vi "Input File Step Iterator.vi"(6 "error in (no error)":errorcluster, 8 "LBCB Input Files":path[](array[path]), 9 "Input File Step Actions":T4) -> (0 "error out":errorcluster, 1 "End of Input File":bool, 2 "Last Step":i32, 3 "Next Step":T1)   [LabVIEW 2009]
uses:
  Input File Step Actions.ctl
  MixedMode/Load Step.ctl
  MixedMode/Messages/Target.ctl
  Data Access Objects/Metadata/LBCB Number.ctl
panel:
  out "Current Step":i32
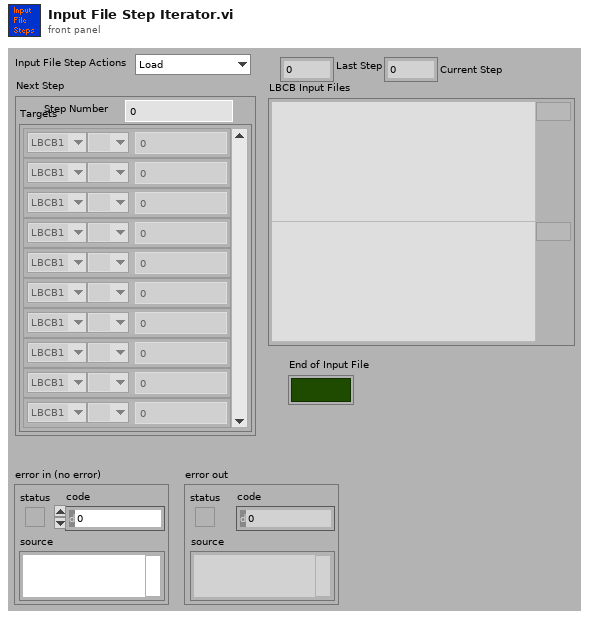
[diagram p1: front panel]
types:
  T1 = typedef "Load Step.ctl" = cluster{"Step Number":u32, "Targets":T2[]}
  T2 = typedef "Target.ctl" = cluster{"LBCB Number":T3, "DOF Vectors":enum16{" ", "Dx", "Dy", "Dz", "Rx", "Ry", "Rz", "Fx", "Fy", "Fz", "Mx", "My", "Mz"}, "Amount":dbl}
  T3 = typedef "LBCB Number.ctl" = enum16{"LBCB1", "LBCB2"}
  T4 = typedef "Input File Step Actions.ctl" = enum16{"Load", "Next Step", "Reset", "Get Step", "Backup"}
  T5 = enum16{"Init", "Set Step", "Set Correction Step", "Set Step String", "Get Step String"}
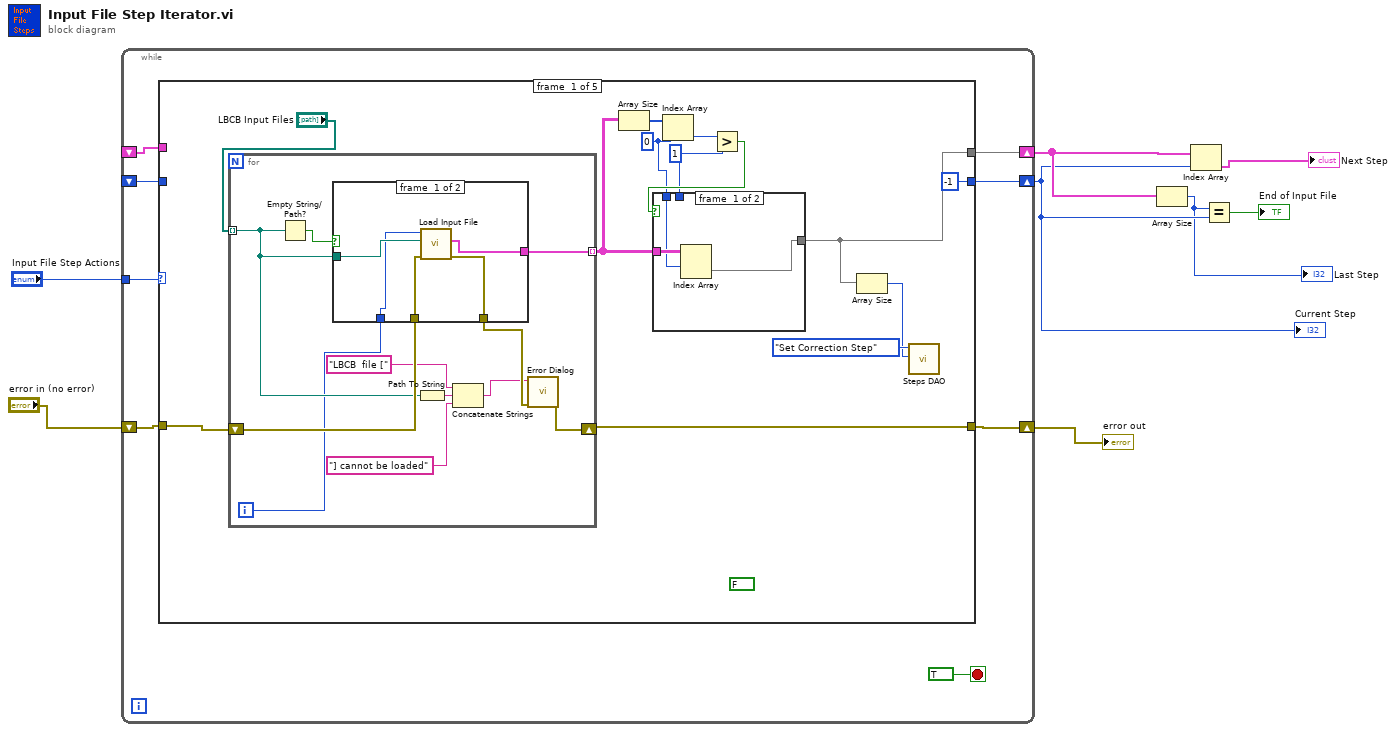
[diagram p0: block diagram]
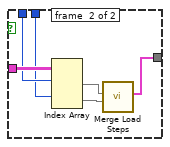
[diagram p2: hidden frame]
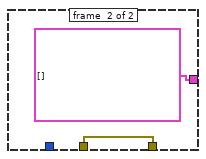
[diagram p3: hidden frame]
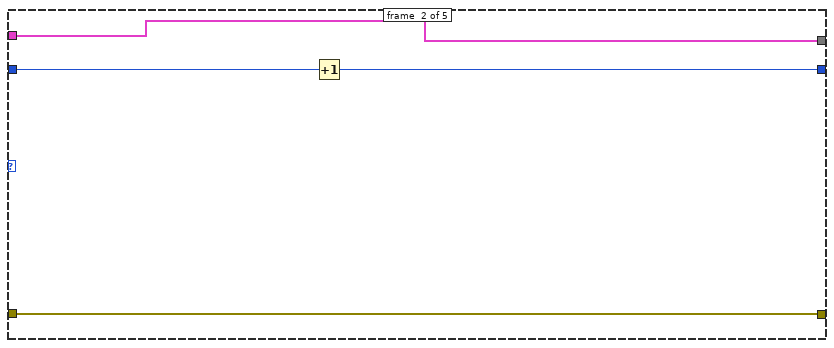
[diagram p4: hidden frame]
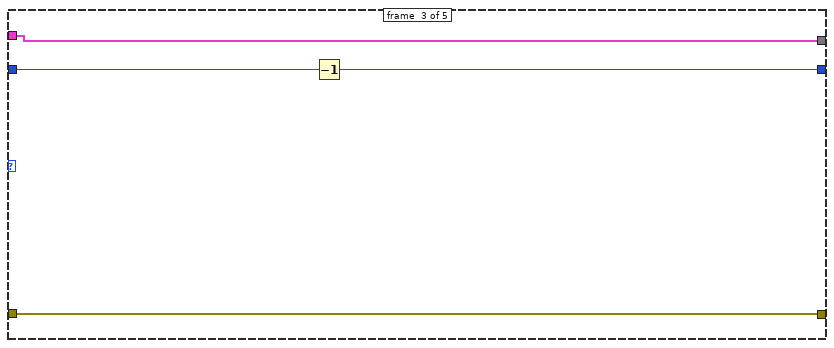
[diagram p5: hidden frame]
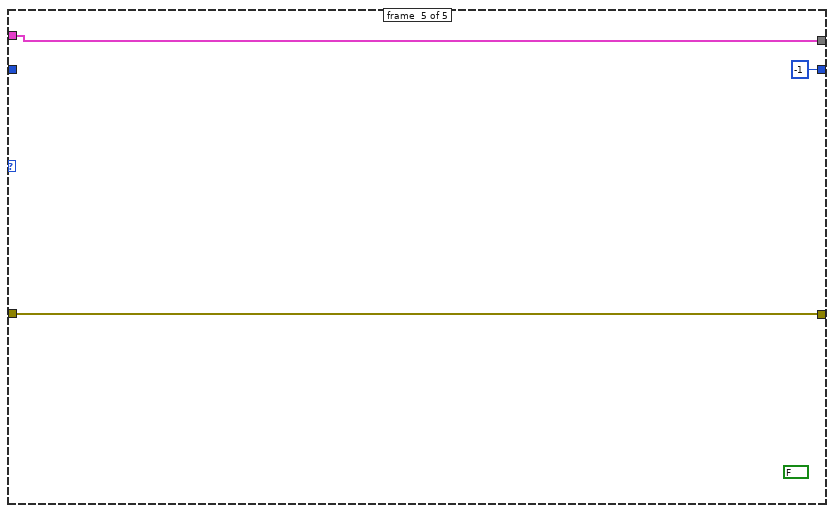
[diagram p7: hidden frame]
diagram:
  n1 = while {
    tunnel: "Input File Step Actions" -> [w15]
    shift-right: [w13] -> w6
    shift-left: "error in (no error)" -> [w14]
    shift-right: [w12] -> w5
    shift-left: _ -> [w10]
    shift-right: [w11] -> w4
    shift-left: _ -> [w9]
    stop <- TRUE stop-if-true
    n2 = case shown="\"Load\"" w15 {
      tunnel: w14 -> [w29 w59 w63 w67 w69]
      tunnel: [w27 w59 w63 w67 w69] -> w13
      tunnel: [w18 w57 w62 w66 w70] -> w12
      tunnel: [-1 w58 w61 w65 -1] -> w11
      tunnel: w10 -> [_ w57 w62 w66 w70]
      tunnel: w9 -> [_ w60 w64 w65 _]
      frame #0 {
        (unwired) FALSE
        w21 = 1 ("y")
        w22 = 0 ("index")
        n3 = for {
          tunnel: "LBCB Input Files" -> [w42] mode=indexing
          shift-right: [w41] -> w27
          shift-left: w29 -> [w48]
          tunnel: [w40] -> w23 mode=indexing
          i -> [w39]
          n4 = Empty String/Path?(string/path=w42) -> (empty?=w49:bool)
          n5 = case shown="False" w49 {
            tunnel: w48 -> [w54 w56]
            tunnel: [w53 w56] -> w46
            tunnel: [w52 T1[] [] ("Load Steps")] -> w40
            tunnel: w42 -> [w51 _]
            tunnel: w39 -> [w50 _]
            frame #0 {
              n6 = call "Load Input File.vi"("error in (no error)"=w54, "Path"=w51, "LBCB Filter"=w50) -> ("error out"=w53:errorcluster, "Load Steps"=w52:T1[])  [unwired: 7 out]
            }
            frame #1 {
            }
          }
          n7 = Path To String(path=w42) -> (string=w47:string)
          n8 = Concatenate Strings("LBCB  file [" ("string"), w47, "] cannot be loaded" ("string")) -> (w45:string)
          n9 = call "Error Dialog.vi"("error in (no error)"=w46, "Message"=w45) -> ("error out"=w41:errorcluster)  [unwired: 9 out]
        }
        n10 = Array Size(array=w23) -> (size(s)=w26:i32[])
        n11 = Index Array(array=w26, index=w22) -> (element=w25:i32)
        n12 = Greater?(x=w25, y=w21) -> (0:w24:bool)
        n13 = case shown="True" w24 {
          tunnel: w23 -> [w32 w38]
          tunnel: w22 -> [w31 w37]
          tunnel: w21 -> [_ w36]
          tunnel: [w30 w33] -> w18
          frame #0 {
            n14 = Index Array(array=w32, index (row)=w31) -> (element=w30:T1[])  [unwired: 1 in]
          }
          frame #1 {
            n15 = Index Array(array=w38, index (row) #1=w37, index (row) #2=w36) -> (element #1=w35:T1[], element #2=w34:T1[])  [unwired: 2 in]
            n16 = call "Merge Load Steps.vi"("Load Steps  In 2"=w34, "Load Steps In"=w35) -> ("Load Steps Out"=w33:T1[])  [unwired: 9 out]
          }
        }
        n17 = Array Size(array=w18) -> (size(s)=w17:i32)
        n18 = call "Steps DAO.vi"("Step In"=w17, "Steps Actions"=T5."Set Correction Step") -> ()  [unwired: 7 in, 3 out]
      }
      frame #1 {
        n19 = Increment(x=w60) -> (x+1=w58:i32)
      }
      frame #2 {
        n20 = Decrement(x=w64) -> (x-1=w61:i32)
      }
      frame #3 {
      }
      frame #4 {
        (unwired) FALSE
      }
    }
  }
  "error out" <- w6
  "Current Step" <- w4
  n21 = Array Size(array=w5) -> (size(s)=w1:i32)
  "Last Step" <- w1
  n22 = Index Array(array=w5, index=w4) -> (element=→"Next Step":T1)
  n23 = Equal?(x=w1, y=w4) -> (x = y?=→"End of Input File":bool)
